vi "Scanner.vi"(8 "error in (no error)":errorcluster, 9 "Range":T1, 10 "Scannable":refnum<class "Scannable.lvclass">, 11 "Scanner.lvclass in":refnum<class "Scanner.lvclass">) -> (0 "error out":errorcluster, 3 "Scanner.lvclass out":refnum<class "Scanner.lvclass">)   [LabVIEW 2017, in "Scanner.lvclass"]
doc: "Protected superclass constructor for Scanner. Make sure you wire your class to the input of this method so it constructs objects with the correct type."
uses:
  Scanner.lvclass
  Instruments/Utility Classes/Scannable/Scannable.lvclass
  Range.ctl
  Scanner.lvclass/Scanner.ctl
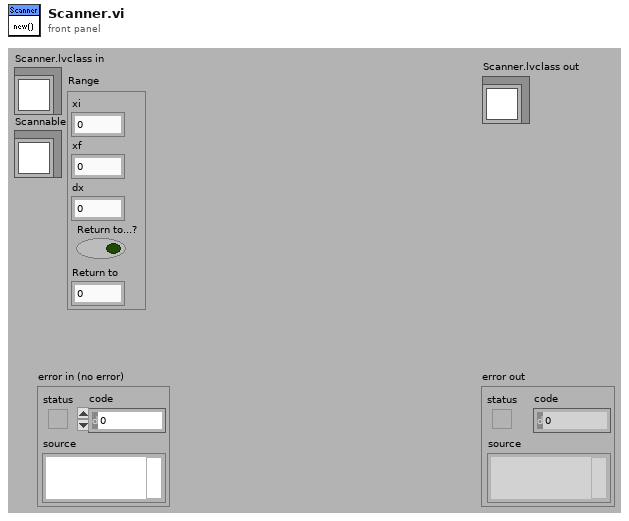
[diagram p1: front panel]
types:
  T1 = typedef "Scanner.lvclass/Range.ctl" = cluster{"xi":dbl, "xf":dbl, "dx":dbl, "Return to...?":bool, "Return to":dbl}
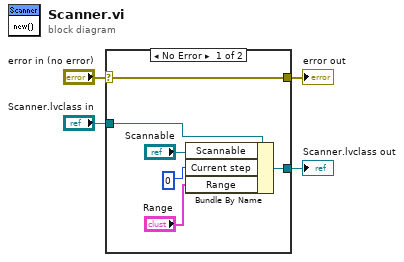
[diagram p0: block diagram]
diagram:
  n1 = case shown="No Error" "error in (no error)" {
    selector: "error in (no error)" -> [w10 w11]
    tunnel: [w10 w11] -> w3
    tunnel: [w8 w12] -> w1
    tunnel: "Scanner.lvclass in" -> [w9 w12]
    frame No Error {
      n2 = Bundle By Name(cluster=w9, "Scannable"="Scannable", "Current step"=u32 0 ("Current Step"), "Range"="Range") -> (w8:refnum<class "Scanner.lvclass">)
    }
    frame Error {
    }
  }
  "error out" <- w3
  "Scanner.lvclass out" <- w1
